vi "Restore Rx IQ Offset Correction Data from File.vi"() -> ()   [LabVIEW 2020]
uses:
  <vilib>/userdefined/Silver/nirio_resource_slv.ctl
  <vilib>/Utility/error.llb/DialogType.ctl
  <instrlib>/niUsrpRio/Config/v1/Host/Public/EEPROM Data Section.ctl
  <vilib>/Utility/file.llb/Read From Spreadsheet File (DBL).vi
  <vilib>/Utility/error.llb/Error Cluster From Error Code.vi
  <vilib>/ErrorRing/Error Ring.xnode
  <instrlib>/niUsrpRio/Config/v1/Host/niUsrpRio Config v1 Host.lvlib
panel:
  in  "USRP RIO Device":T1="Select USRP RIO Device"
  # "Select the USRP RIO device on which you want to load the correction data"
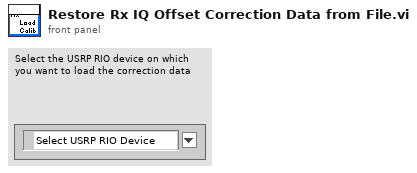
[diagram p1: front panel]
types:
  T1 = typedef "nirio_resource_slv.ctl" = tag
  T2 = typedef "niUsrpRio Config v1 Host.lvlib/EEPROM Data Section.ctl" = enum16{"Factory Data", "User Data"}
  T3 = typedef "DialogType.ctl" = u16
  T4 = typedef "niUsrpRio Config v1 Host.lvlib/niUsrpRio Session.ctl" = cluster{"FPGA Interface":refnum<k20>, "RIO Interface Number":u32, "Data Clock Rate":u32, "FPGA Data Clock Rate":u32, "Global Settings Register Bus":T5, "Radio 0 Settings Register Bus":T5, "Radio 1 Settings Register Bus":T5, "Radio Settings Bus Semaphore":T6, "DB Queues":T7[], "Characterization Data Valid?":bool, "EEPROM Header":T8, "Device Data Header":T9, "EEPROM Characterization Header":T10, "Characterization Data":T11[], "FPGA Current Version":u32, "FPGA Oldest Compatible Version":u32, "Fixed Logic Current Version":u32, "Fixed Logic Oldest Compatible Version":u32, "FPGA Radio Settings Bus Current Version":u32, "FPGA Radio Settings Bus Oldest Compatible Version":u32, "FPGA Board Config Current Version":u32, "FPGA Board Config Oldest Compatible Version":u32, "Daughterboard Clock Rate":u32, "daughterboard configuration session handles":u64[]}
  T5 = typedef "niInstr Register Bus v0 Host.lvlib/Register Bus Session.ctl" = refnum<queue>
  T6 = typedef "Semaphore RefNum" = refnum<k1>
  T7 = typedef "niUsrpRio Config v1 Host.lvlib/DB Queue Reference.ctl" = refnum<queue>
  T8 = typedef "niUsrpRio Config v1 Host.lvlib/EEPROM Header.ctl" = cluster{"Checksum":u32, "Product Code":u16, "Hardware Current Version":u16, "Hardware Oldest Compatible Version":u16, "EEPROM Map Current Version":u16, "EEPROM Map Oldest Compatible Version":u16, "User Password":string, "Pointer to Factory Header":u32, "Pointer to User Header":u32, "Recommended Interval":u16, "Number of Reserved Bytes":i32, "Number of Daughterboards":u8, "Daughterboard IDs":u16[], "Daughterboard Serial Numbers":string[]}
  T9 = typedef "niUsrpRio Config v1 Host.lvlib/EEPROM Device Data Header.ctl" = cluster{"Checksum":u32, "Number of Channels":u8, "Number of Gain Settings":u16[], "Pointer to Characterization Data":u32[], "Number of Reserved Bytes":i32, "Number of Frequencies":u16[]}
  T10 = typedef "niUsrpRio Config v1 Host.lvlib/EEPROM Characterization Header.ctl" = cluster{"Checksum":u32, "Date":timestamp, "Temperature":sgl, "Misc. Info":string, "Pointer to Device Data Header":u32, "Number of Reserved Bytes":i32}
  T11 = typedef "niUsrpRio Config v1 Host.lvlib/Characterization Data.ctl" = cluster{"Gains[dB]":dbl[], "Frequencies [Hz]":dbl[], "IQ Imbalance Table":T12[], "Measured Gains[dB]":dbl[][]}
  T12 = typedef "niUsrpRio Config v1 Host.lvlib/IQ Imbalance.ctl" = cluster{"Gain Imbalance [linear]":dbl, "Phase Imbalance [radians]":dbl, "Offset":cdb}
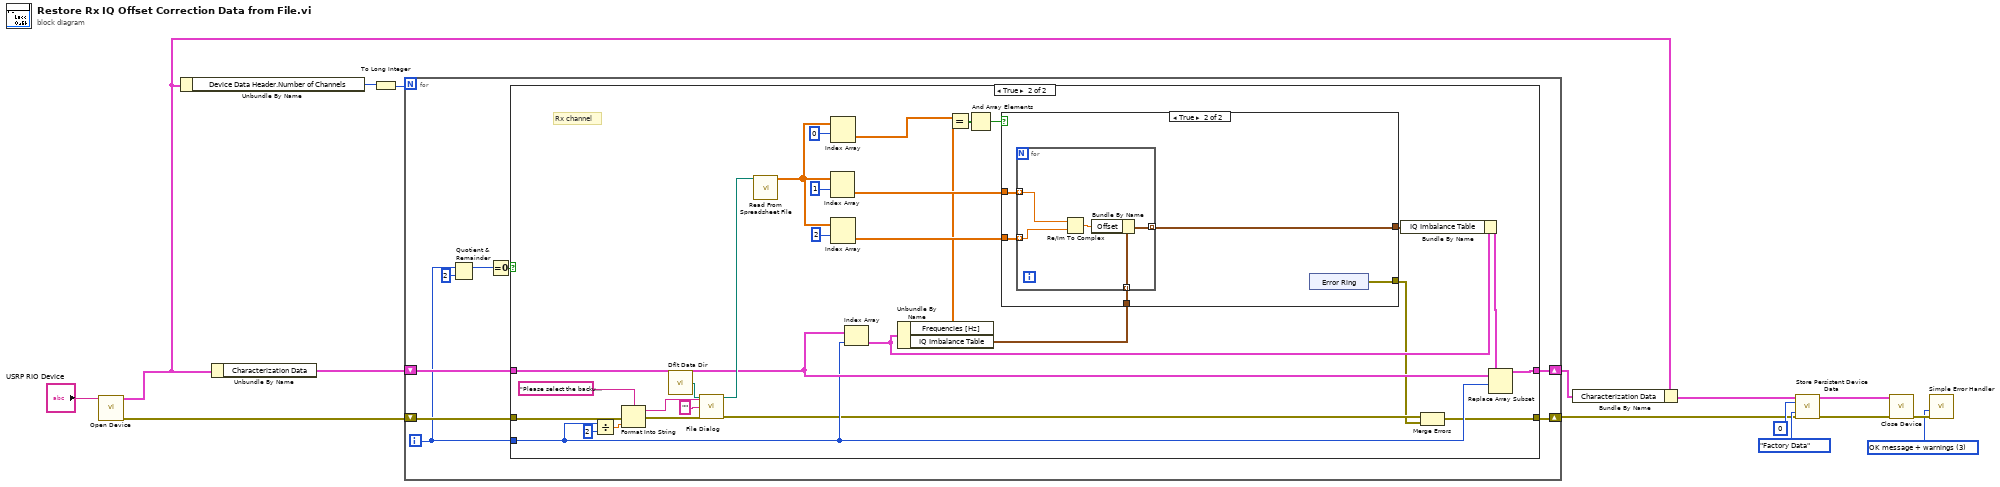
[diagram p0: block diagram]
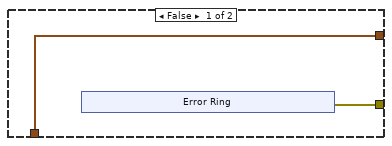
[diagram p3: hidden frame]
diagram:
  w11 = T3 3 items=["no dialog", "OK message", "continue or stop message", "OK message + warnings", "continue/stop + warnings"] ("type of dialog (OK msg:1)")
  n1 = call "Open Device.vi"("USRP RIO device"="USRP RIO Device") -> ("niUsrpRio Session (out)"=w10:T4, "error out"=w8:errorcluster)  [unwired: 13 in]
  n2 = Unbundle By Name(w10) -> ("Device Data Header.Number of Channels"=w5:u8)
  n3 = Unbundle By Name(w10) -> ("Characterization Data"=w7:T11[])
  n4 = To Long Integer(number=w5) -> (32bit integer=w4:i32)
  n5 = for {
    N: w4 -> [_]
    shift-right: [w23] -> w6
    shift-left: w7 -> [w22]
    shift-right: [w20] -> w1
    shift-left: w8 -> [w21]
    i -> [w16]
    n6 = Quotient & Remainder(x=w16, y=2) -> (x-y*floor(x/y)=w18:i32)  [unwired: 1 out]
    n7 = Equal To 0?(x=w18) -> (x = 0?=w17:bool)
    n8 = case shown="TRUE" w17 {
      tunnel: [w25 w50] -> w23
      tunnel: w22 -> [w25 w49]
      tunnel: w21 -> [w24 w28]
      tunnel: [w24 w30] -> w20
      tunnel: w16 -> [_ w46]
      frame False {
        # "There is no information saved for Tx"
        # "Tx channel"
      }
      frame True {
        # "Rx channel"
        n9 = Divide(x=w46, y=2) -> (x/y=w47:dbl)
        n10 = Format Into String(format string="Please select the backup data file for Rx Channel  %d" ("prompt"), error in=w28, w47) -> (resulting string=w51:string, error out=w29:errorcluster)  [unwired: 1 in]
        n11 = call <vilib>:"Dflt Data Dir.vi"() -> ("App:Default Data Directory"=w48:path)
        n12 = call "File Dialog"("start path"=w48, "prompt"=w51, "default name"="", "error in"=w29) -> ("selected path"=w53:path, "error out"=w27:errorcluster)  [unwired: 8 in, 2 out]
        n13 = call-poly <vilib>:"Read From Spreadsheet File.vi"("file path (dialog if empty)"=w53) -> ("all rows"=w42:dbl[][])  [unwired: 6 in, 4 out]
        n14 = Index Array(array=w42, index (row)=1) -> (element=w39:dbl[])  [unwired: 1 in]
        n15 = Index Array(array=w42, index (row)=0) -> (element=w33:dbl[])  [unwired: 1 in]
        n16 = Index Array(array=w42, index (row)=2) -> (element=w40:dbl[])  [unwired: 1 in]
        n17 = Index Array(array=w49, index=w46) -> (element=w36:T11)
        n18 = Unbundle By Name(w36) -> ("Frequencies [Hz]"=w34:dbl[], "IQ Imbalance Table"=w35:T12[])
        n19 = Equal?(x=w33, y=w34) -> (x = y?=w32:bool[])
        n20 = And Array Elements(Boolean array=w32) -> (logical AND=w31:bool)
        n21 = case shown="TRUE" w31 {
          tunnel: w40 -> [_ w66]
          tunnel: w39 -> [_ w65]
          tunnel: [w56 w64] -> w38
          tunnel: w35 -> [w56 w63]
          tunnel: [w55 w62] -> w26
          frame False {
            n22 = xnode "Error Ring"() -> ("エラー出力"=w55:errorcluster)
          }
          frame True {
            n23 = for {
              tunnel: w66 -> [w69] mode=indexing
              tunnel: w65 -> [w70] mode=indexing
              tunnel: [w72] -> w64 mode=indexing
              tunnel: w63 -> [w71] mode=indexing
              n24 = Re/Im To Complex(1:w69, 2:w70) -> (0:w68:cdb)
              n25 = Bundle By Name(cluster=w71, "Offset"=w68) -> (w72:T12)
            }
            n26 = xnode "Error Ring"() -> ("エラー出力"=w62:errorcluster)
          }
        }
        n27 = Bundle By Name(cluster=w36, "IQ Imbalance Table"=w38) -> (w37:T11)
        n28 = Merge Errors(w27, w26) -> (w30:errorcluster)
        n29 = Replace Array Subset(array=w49, new element=w37, index=w46) -> (w50:T11[])
      }
    }
  }
  n30 = Bundle By Name(cluster=w10, "Characterization Data"=w6) -> (w9:T4)
  n31 = call <instrlib>:"Store Persistent Device Data.vi"("niUsrpRio session"=w9, "offset"=u32 0, "EEPROM Data Section"=EEPROM_Data_Section."Factory Data", "error in"=w1) -> ("niUsrpRio session (out)"=w14:T4, "error out"=w13:errorcluster)  [unwired: 10 in]
  n32 = call "Close Device.vi"("niUsrpRio Session"=w14, "error in"=w13) -> ("error out"=w12:errorcluster)  [unwired: 13 in]
  n33 = call <vilib>:"Simple Error Handler.vi"("type of dialog (OK msg:1)"=w11, "error in (no error)"=w12) -> ()  [unwired: 3 in, 5 out]
